vi "ChannelList_GetNames.vi"(8 "error in (no error)":errorcluster, 11 "OXY_SCPI Reseource In":refnum<visa-resource-name>) -> (0 "error out":errorcluster, 1 "communication_data":T1, 2 "Channels":cluster{"ID":string, "Name":string}[](array[cluster]), 3 "OXY_SCPI Reseource Out":refnum<visa-resource-name>)   [LabVIEW 2020, in "OXYGEN_Datastream.lvlib"]
doc: "Queries the name and ids of all channels."
uses:
  OXYGEN_Datastream.lvlib
  TypeDefs/Cluster_RawCommData.ctl
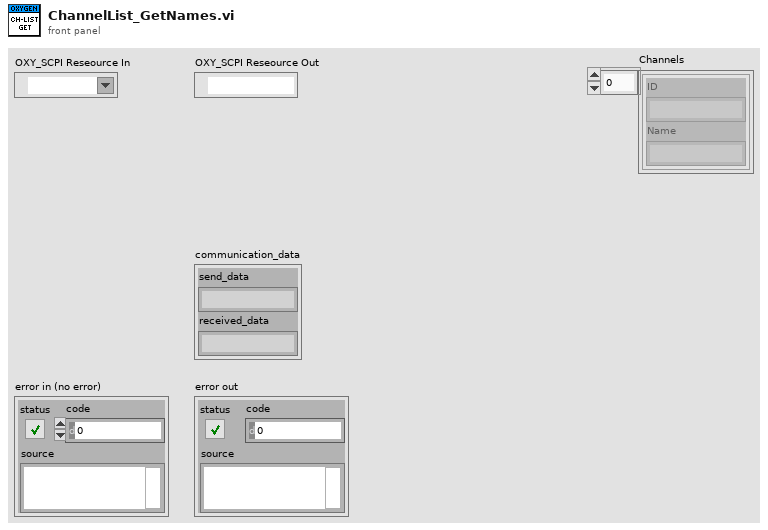
[diagram p1: front panel]
types:
  T1 = typedef "OXYGEN_Datastream.lvlib/Cluster_RawCommData.ctl" = cluster{"send_data":string, "received_data":string}
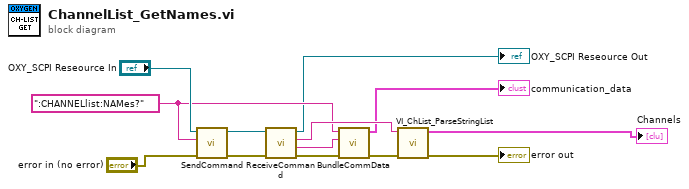
[diagram p0: block diagram]
diagram:
  w5 = ":CHANNELlist:NAMes?"
  n1 = call "SendCommand.vi"("error in (no error)"="error in (no error)", "String to Send"=w5, "OXY_SCPI Reseource In"="OXY_SCPI Reseource In") -> ("error out"=w13:errorcluster, "OXY_SCPI Reseource Out"=w12:refnum<visa-resource-name>)  [unwired: 7 in]
  n2 = call "ReceiveCommand.vi"("error in (no error)"=w13, "OXY_SCPI Reseource In"=w12) -> ("error out"=w11:errorcluster, "received Data with Header"=w7:string, "received Data"=w6:string, "OXY_SCPI Reseource Out"=→"OXY_SCPI Reseource Out":refnum<visa-resource-name>)  [unwired: 6 in]
  n3 = call "BundleCommData.vi"("error in (no error)"=w11, "received_data"=w7, "send_data"=w5) -> ("error out"=w10:errorcluster, "communication_data"=→"communication_data":T1)  [unwired: 7 in]
  n4 = call "VI_ChList_ParseStringList.vi"("error in (no error)"=w10, "ChList_RawString"=w6) -> ("error out"=→"error out":errorcluster, "Channel List"=→"Channels":cluster{"ID":string, "Name":string}[])  [unwired: 8 in]
